vi "RichToFlatcif_manager_Error.vi"(5 "OutputClusterType":T1, 11 "InputCluster":T2) -> (3 "OutputCluster":T1)   [LabVIEW 2021, in "CIF_Manager_client.lvlib"]
uses:
  CIF_Manager_client.lvlib
  cif_manager_Error.ctl
  cif_manager_Error_Flat.ctl
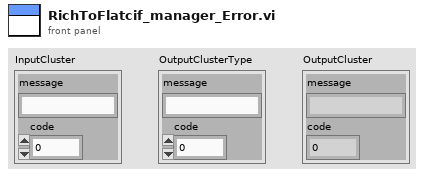
[diagram p1: front panel]
types:
  T1 = typedef "CIF_Manager_client.lvlib/cif_manager_Error_Flat.ctl" = cluster{"message":string, "code":i32}
  T2 = typedef "CIF_Manager_client.lvlib/cif_manager_Error.ctl" = cluster{"message":string, "code":i32}
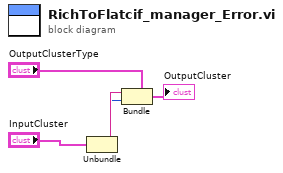
[diagram p0: block diagram]
diagram:
  n1 = Unbundle "Unbundle"("InputCluster") -> ("message"=w2:string, "code"=w1:i32)
  n2 = Bundle "Bundle"(cluster="OutputClusterType", "message"=w2, "code"=w1) -> (→"OutputCluster":T1)
